vi "Extract uService List from CSV.vi"(8 "error in (no error)":errorcluster, 9 "Guardian ID":string, 10 "CSV table":string[][](array[string])) -> (0 "error out":errorcluster, 2 "uS array":string[](array[string]))   [LabVIEW 2026, in "TALOS.lvlib" / "Guardian.lvlib" / "Guardian.lvclass"]
uses:
  Guardian.lvclass
  6b7e15ba-f9cb-416d-a90f-28e9ee05c1ec.vi
  11cba1b9-d4f5-4b07-bd60-c0254bd7e6eb.vi
  3e5d1c94-8dd5-40b1-9352-efdc3e985fe4.vi
  <userlib>/_OpenG.lib/string/string.llb/Trim Whitespace (String)__ogtk.vi
  <vilib>/Comparison/Equal/Equal Functor/Equal Functor.lvclass
  <userlib>/_OpenG.lib/string/string.llb/openg_string.lvlib
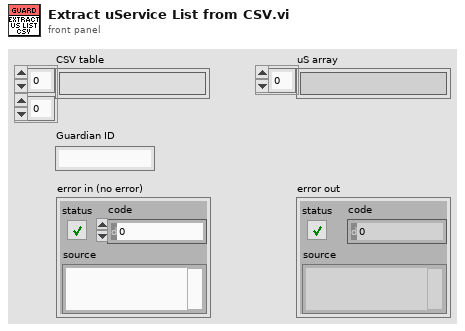
[diagram p1: front panel]
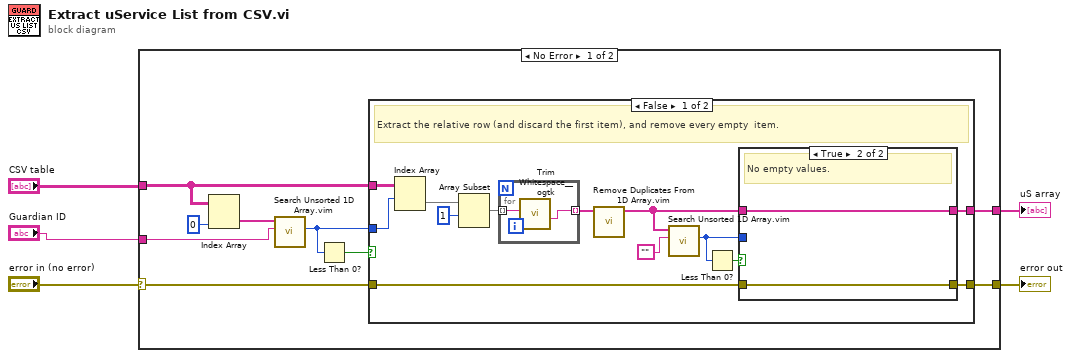
[diagram p0: block diagram]
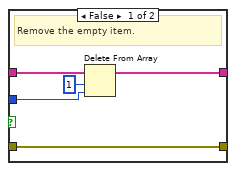
[diagram p2: hidden frame]
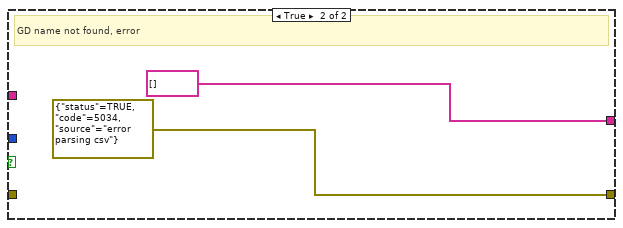
[diagram p3: hidden frame]
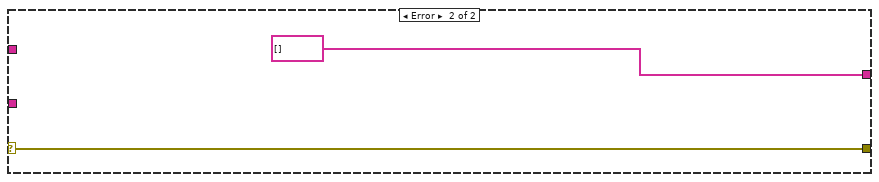
[diagram p4: hidden frame]
diagram:
  n1 = case shown="No Error" "error in (no error)" {
    selector: "error in (no error)" -> [w7 w40]
    tunnel: "CSV table" -> [w11 _]
    tunnel: [w8 w40] -> w5
    tunnel: [w9 string[] []] -> w4
    tunnel: "Guardian ID" -> [w6 _]
    frame No Error {
      n2 = Index Array(array=w11, index (col)=0 ("disabled index (col)")) -> (element=w13:string[])  [unwired: 1 in]
      n3 = call "Search Unsorted 1D Array.vim"("element"=w6, "unsorted 1D array"=w13) -> ("index of element"=w10:i32)  [unwired: 9 in]
      n4 = Less Than 0?(x=w10) -> (x < 0?=w12:bool)
      n5 = case shown="False" w12 {
        tunnel: w11 -> [w27 _]
        tunnel: w10 -> [w26 _]
        tunnel: [w18 string[] []] -> w9
        tunnel: [w19 errorcluster {"status"=TRUE, "code"=5034, "source"="error parsing csv"} ("error IO")] -> w8
        tunnel: w7 -> [w20 _]
        frame False {
          # "Extract the relative row (and discard the first item), and remove every empty  item."
          n6 = Index Array(array=w27, index (row)=w26) -> (element=w25:string[])  [unwired: 1 in]
          n7 = Array Subset(array=w25, index=1) -> (w17:string[])  [unwired: 1 in]
          n8 = for {
            tunnel: w17 -> [w29] mode=indexing
            tunnel: [w28] -> w16 mode=indexing
            n9 = call-poly <userlib>:"Trim Whitespace__ogtk.vi"("String in"=w29) -> ("String out"=w28:string)  [unwired: 6 in]
          }
          n10 = call "Remove Duplicates From 1D Array.vim"("array"=w16) -> ("array with duplicates removed"=w15:string[])  [unwired: 10 in]
          n11 = call "Search Unsorted 1D Array.vim"("element"="", "unsorted 1D array"=w15) -> ("index of element"=w21:i32)  [unwired: 9 in]
          n12 = Less Than 0?(x=w21) -> (x < 0?=w22:bool)
          n13 = case shown="True" w22 {
            tunnel: w21 -> [w33 _]
            tunnel: w15 -> [w34 w36]
            tunnel: [w31 w36] -> w18
            tunnel: w20 -> [w30 w35]
            tunnel: [w30 w35] -> w19
            frame False {
              # "Remove the empty item."
              n14 = Delete From Array(array=w34, length=1, index=w33) -> (array with subset deleted=w31:string[])  [unwired: 1 out]
            }
            frame True {
              # "No empty values."
            }
          }
        }
        frame True {
          # "GD name not found, error"
        }
      }
    }
    frame Error {
    }
  }
  "error out" <- w5
  "uS array" <- w4
